vi "_ASIC_TEST_enlace.vi"(8 "error in":errorcluster, 11 "ftHandle_in":u32) -> (0 "error out":errorcluster, 3 "ftHandle_out":u32)   [LabVIEW 2009]
panel:
  out "Scaler 3 (20,21)":u16 format="%04x"
  out "Scaler 2 (18,19)":u16 format="%04x"
  out "Scaler 1 (16,17)":u16 format="%04x"
  out "Lectura asic (14,15)":u16 format="%04x"
  out "Vent. Sacaler (11,12,13)":u32 format="%06x"
  out "Periodo VGa (9,10)":u16 format="%04x"
  out "Pulse VGa (7,8)":u16 format="%04x"
  out "Ganacia VGA (6)":u8 format="%02x"
  out "adc (4,5)":u16 format="%04x"
  out "Asic (1,2,3)":u32 format="%06x"
  out "DIR 0 (CONFIG)":bool[](array[boolean])
  out "ERROR":bool
  out "DAC_IB":bool[](array[boolean])
  out "BUFF_ENA":bool
  out "LVDS_ENA1":bool
  out "LVDS_ENA0":bool
  out "MUX_ENA":string
  out "MUX_ENA#":i32
  out "IN 0":bool[](array[boolean])
  out "IN 6":bool[](array[boolean])
  out "IN 5":bool[](array[boolean])
  out "IN 4":bool[](array[boolean])
  out "IN 3":bool[](array[boolean])
  out "IN 2":bool[](array[boolean])
  out "IN 1":bool[](array[boolean])
  out "DAC_MUX#":i32
  out "DAC_MUX":string
  out "TH5":u16 format="%010b"
  out "TH4":u16 format="%010b"
  out "TH3":u16 format="%010b"
  out "TH2":u16 format="%010b"
  out "TH1":u16 format="%010b"
  out "TH0":u16 format="%010b"
  # "start vent. sca\nescribir ganancia\nactualizar pulso\nenable pulso\nstart tx asic\nreset asic\nescribir adc"
  # "Control_byte\nNum bit        Función\n0            \"Escribir\" ADC\n1                      \"INIT_R\" ASIC (reset)\n2                      \"start_tx\" ASIC para configuración ASIC\n3                      \"enable\" para el pulso\n4                      \"actualizar\" para el pulso\n5                      \"Escribir_ganancia\" para configuración ganancia\n6                      \"start\" para apertura ventana temportal scalers"
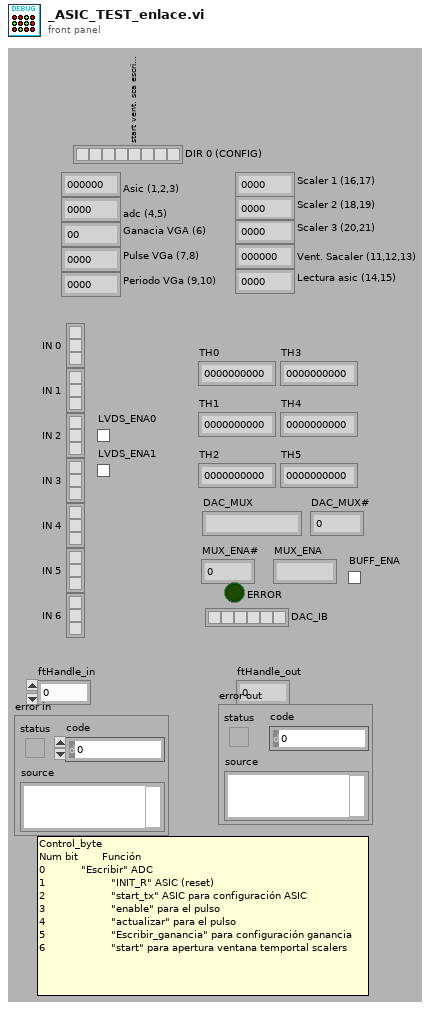
[diagram p1: front panel]
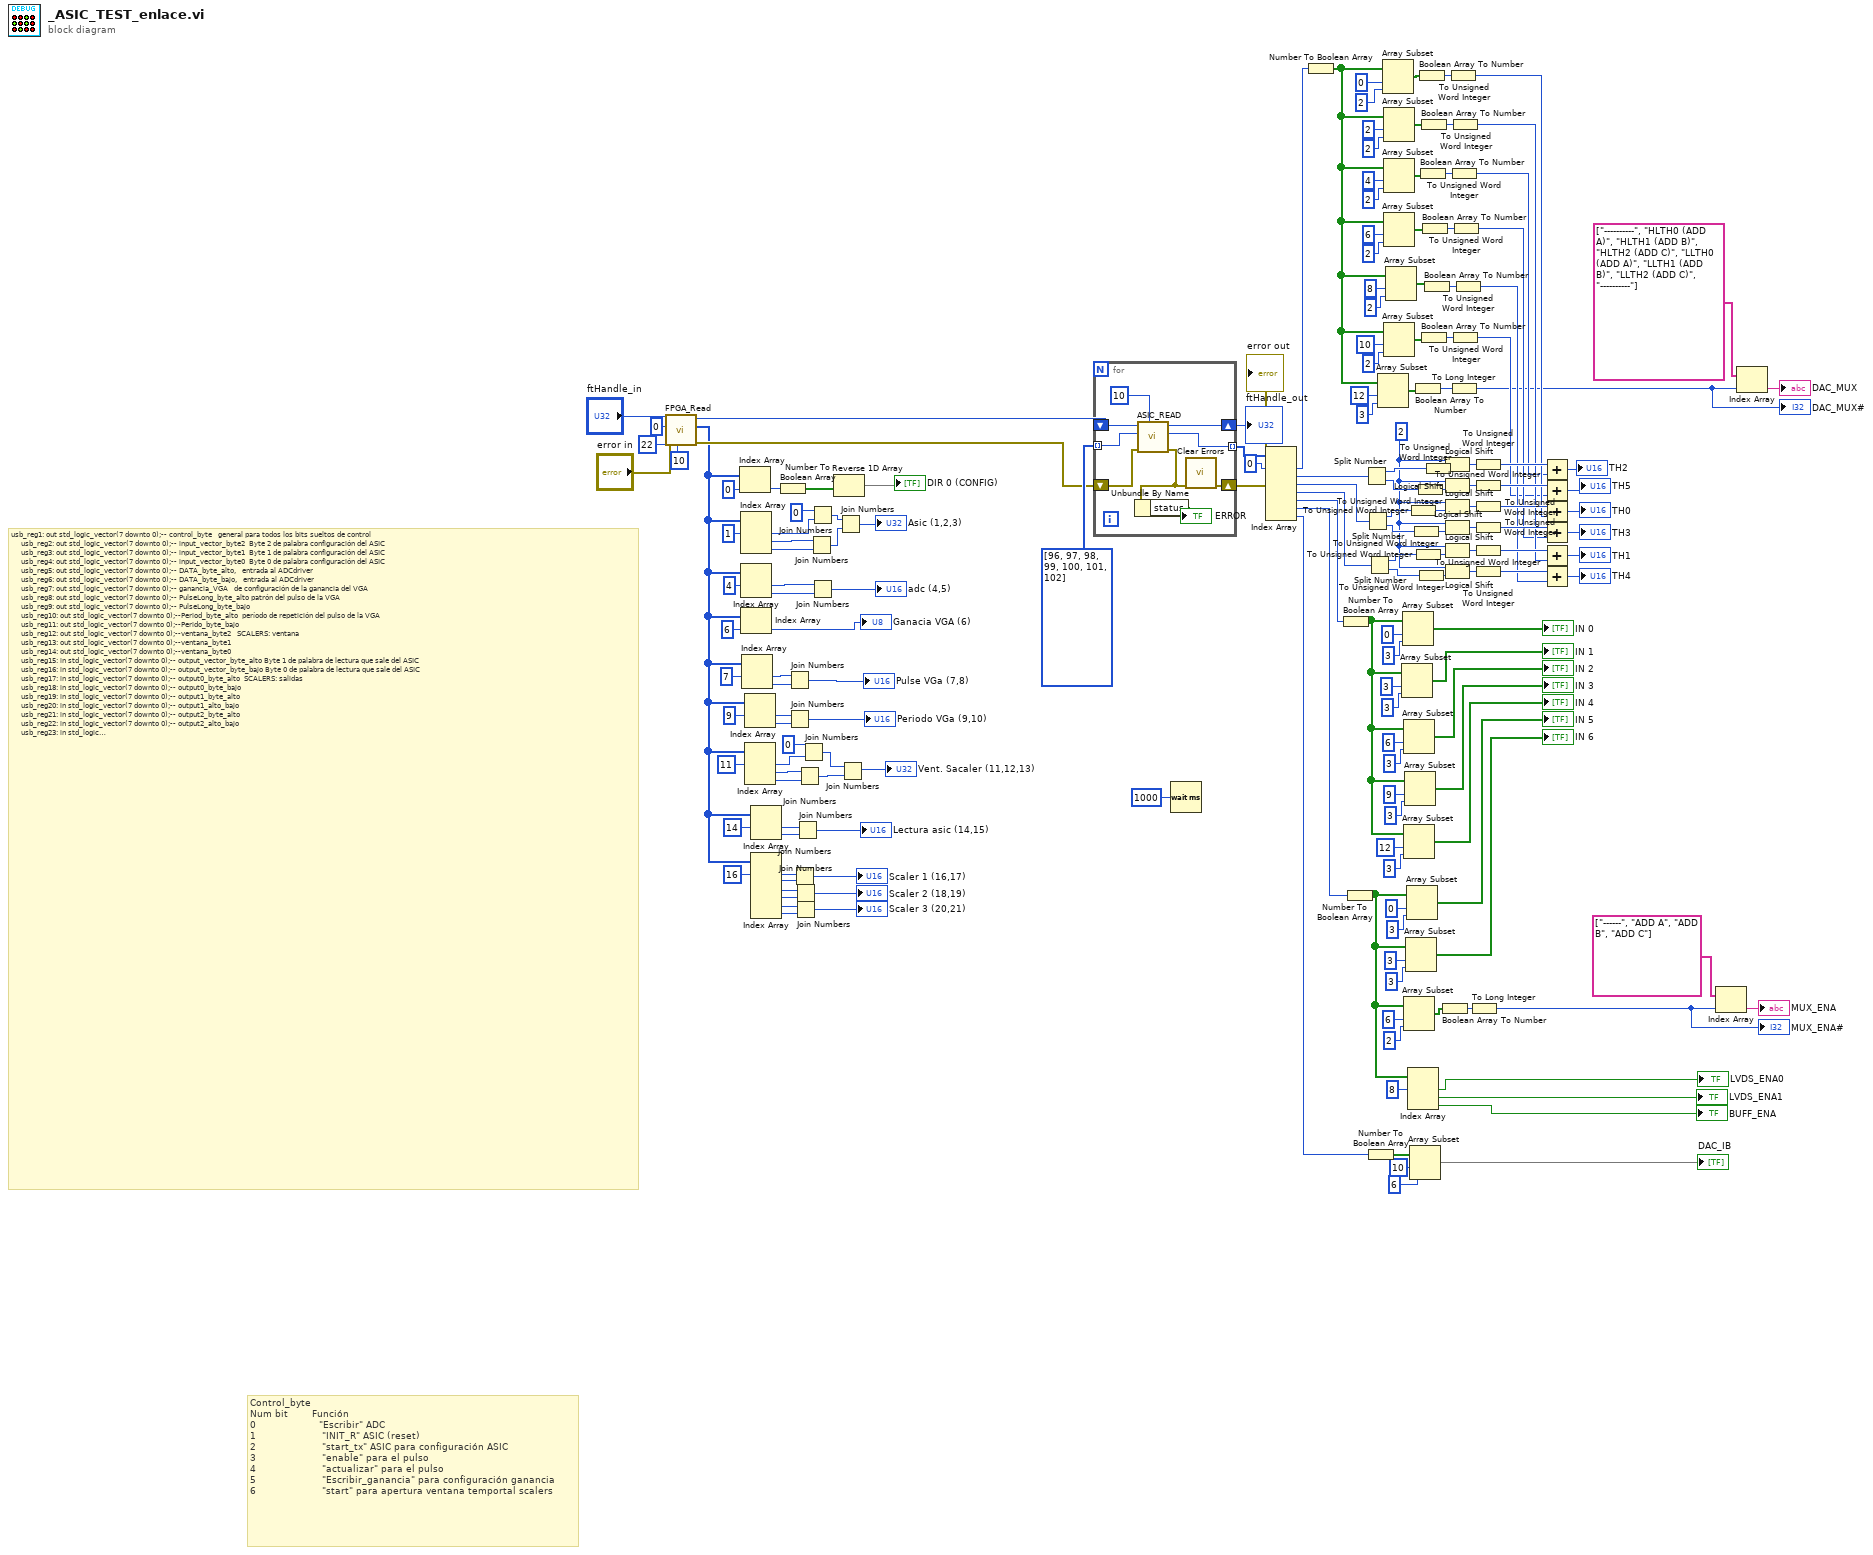
[diagram p0: block diagram]
diagram:
  w165 = i8 2 ("y")
  # "Control_byte\nNum bit        Función\n0                     \"Escribir\" ADC\n1                      \"INIT_R\" ASIC (reset)\n2                      \"start_tx\" ASIC para configuración ASIC\n3                      \"enable\" para el pulso\n4                      \"actualizar\" para el pulso\n5                      \"Escribir_ganancia\" para configuración ganancia\n6                      \"start\" para apertura ventana temportal scalers"
  # "usb_reg1: out std_logic_vector(7 downto 0);-- control_byte\t\t\tgeneral para todos los bits sueltos de control\n\t\t\t  usb_reg2: out std_logic_vector(7 downto 0);-- input_vector_byte2 \tByte 2 de palabra configuración del ASIC\n\t\t\t  usb_reg3: out std_logic_vector(7 downto 0);-- input_vector_byte1 \tByte 1 de palabra configuración del ASIC\n\t\t\t  usb_reg4: out std_logic_vector(7 downto 0);-- input_vector_byte0 \tByte 0 de palabra configuración del ASIC\n\t\t\t  usb_reg5: out std_logic_vector(7 downto 0);-- DATA_byte_alto, \t\tentrada al ADCdriver\n\t\t\t  usb_reg6: out std_logic_vector(7 downto 0);-- DATA_byte_bajo, \t\tentrada al ADCdriver\n\t\t\t  usb_reg7: out std_logic_vector(7 downto 0);-- ganancia_VGA\t\t\tde configuración de la ganancia del VGA\n\t\t\t  usb_reg8: out std_logic_vector(7 downto 0);-- PulseLong_byte_alto\tpatrón del pulso de la VGA\n\t\t\t  usb_reg9: out std_logic_vector(7 downto 0);-- PulseLong_byte_bajo\n\t\t\t  usb_reg10: out std_logic_vector(7 downto 0);--Period_byte_alto\t\tperíodo de repetición del pulso de la VGA\n\t\t\t  usb_reg11: out std_logic_vector(7 downto 0);--Perido_byte_bajo\n\t\t\t  usb_reg12: out std_logic_vector(7 downto 0);--ventana_byte2\t\t\tSCALERS: ventana\n\t\t\t  usb_reg13: out std_logic_vector(7 downto 0);--ventana_byte1\t\n\t\t\t  usb_reg14: out std_logic_vector(7 downto 0);--ventana_byte0\n\t\t\t  usb_reg15: in std_logic_vector(7 downto 0);-- output_vector_byte_alto\tByte 1 de palabra de lectura que sale del ASIC\n\t\t\t  usb_reg16: in std_logic_vector(7 downto 0);-- output_vector_byte_bajo\tByte 0 de palabra de lectura que sale del ASIC\n\t\t\t  usb_reg17: in std_logic_vector(7 downto 0);-- output0_byte_alto\t\tSCALERS: salidas\n\t\t\t  usb_reg18: in std_logic_vector(7 downto 0);-- output0_byte_bajo\n\t\t\t  usb_reg19: in std_logic_vector(7 downto 0);-- output1_byte_alto\n\t\t\t  usb_reg20: in std_logic_vector(7 downto 0);-- output1_alto_bajo \n\t\t\t  usb_reg21: in std_logic_vector(7 downto 0);-- output2_byte_alto \n\t\t\t  usb_reg22: in std_logic_vector(7 downto 0);-- output2_alto_bajo \n\t\t\t  usb_reg23: in std_logic_vector(7 downto 0);-- para el canal_0 del ADCdriver\n\t\t\t  usb_reg24: in std_logic_vector(7 downto 0);\n\t\t\t  usb_reg25: in std_logic_vector(7 downto 0);-- para el canal_1 del ADCdriver\n\t\t\t  usb_reg26: in std_logic_vector(7 downto 0);\n\t\t\t  usb_reg27: in std_logic_vector(7 downto 0);-- para el canal_2 del ADCdriver\n\t\t\t  usb_reg28: in std_logic_vector(7 downto 0);\n\t\t\t  usb_reg29: in std_logic_vector(7 downto 0);-- para el canal_3 del ADCdriver\n\t\t\t  usb_reg30: in std_logic_vector(7 downto 0);\n\t\t\t  usb_reg31: in std_logic_vector(7 downto 0);-- para el canal_4 del ADCdriver\n\t\t\t  usb_reg32: in std_logic_vector(7 downto 0);\n\t\t\t  usb_reg33: in std_logic_vector(7 downto 0);-- para el canal_5 del ADCdriver\n\t\t\t  usb_reg34: in std_logic_vector(7 downto 0);\n\t\t\t  usb_reg35: in std_logic_vector(7 downto 0);-- para el canal_6 del ADCdriver\n\t\t\t  usb_reg36: in std_logic_vector(7 downto 0);\n\t\t\t  usb_reg37: in std_logic_vector(7 downto 0);-- para el canal_7 del ADCdriver\n\t\t\t  usb_reg38: in std_logic_vector(7 downto 0);\n\t\t\t  usb_reg39: in std_logic_vector(7 downto 0);-- para el canal_8 del ADCdriver\n\t\t\t  usb_reg40: in std_logic_vector(7 downto 0);\n\t\t\t  usb_reg41: in std_logic_vector(7 downto 0);-- para el canal_9 del ADCdriver\n\t\t\t  usb_reg42: in std_logic_vector(7 downto 0);\n\t\t\t  usb_reg43: in std_logic_vector(7 downto 0);-- para el canal_10 del ADCdriver\n\t\t\t  usb_reg44: in std_logic_vector(7 downto 0)--;"
  n1 = call "FPGA_Read.vi"("Espera acceso USB"=u32 10, "error in"="error in", "Numero Bytes"=u8 22, "Dirección base"=u8 0, "ftHandle_in"="ftHandle_in") -> ("error out"=w56:errorcluster, "lpBuffer_out"=w15:u8[], "ftHandle_out"=w58:u32)  [unwired: 2 in, 2 out]
  n2 = Index Array(array=w15, index=0) -> (element=w37:u8)
  n3 = Index Array(array=w15, index #1=1 ("index")) -> (element #1=w32:u8, element #2=w33:u8, element #3=w34:u8)  [unwired: 2 in]
  n4 = Index Array(array=w15, index #1=4 ("index")) -> (element #1=w31:u8, element #2=w30:u8)  [unwired: 1 in]
  n5 = Index Array(array=w15, index=6) -> (element=→"Ganacia VGA (6)":u8)
  n6 = Index Array(array=w15, index #1=7 ("index")) -> (element #1=w24:u8, element #2=w25:u8)  [unwired: 1 in]
  n7 = Index Array(array=w15, index #1=9 ("index")) -> (element #1=w22:u8, element #2=w23:u8)  [unwired: 1 in]
  n8 = Index Array(array=w15, index #1=11 ("index")) -> (element #1=w18:u8, element #2=w16:u8, element #3=w17:u8)  [unwired: 2 in]
  n9 = Index Array(array=w15, index #1=14 ("index")) -> (element #1=w14:u8, element #2=w13:u8)  [unwired: 1 in]
  n10 = Index Array(array=w15, index #1=16 ("index")) -> (element #1=w11:u8, element #2=w10:u8, element #3=w8:u8, element #4=w7:u8, element #5=w6:u8, element #6=w5:u8)  [unwired: 5 in]
  n11 = Number To Boolean Array(number=w37) -> (Boolean array=w39:bool[])
  n12 = Join Numbers(hi=w24, lo=w25) -> ((hi.lo)=→"Pulse VGa (7,8)":u16)
  n13 = Join Numbers(hi=w22, lo=w23) -> ((hi.lo)=→"Periodo VGa (9,10)":u16)
  n14 = Join Numbers(hi=w11, lo=w10) -> ((hi.lo)=→"Scaler 1 (16,17)":u16)
  n15 = Join Numbers(hi=w8, lo=w7) -> ((hi.lo)=→"Scaler 2 (18,19)":u16)
  n16 = Join Numbers(hi=w6, lo=w5) -> ((hi.lo)=→"Scaler 3 (20,21)":u16)
  n17 = Join Numbers(hi=w14, lo=w13) -> ((hi.lo)=→"Lectura asic (14,15)":u16)
  n18 = Join Numbers(hi=w16, lo=w17) -> ((hi.lo)=w48:u16)
  n19 = Join Numbers(hi=u8 0, lo=w18) -> ((hi.lo)=w42:u16)
  n20 = Join Numbers(hi=w33, lo=w34) -> ((hi.lo)=w53:u16)
  n21 = Join Numbers(hi=u8 0, lo=w32) -> ((hi.lo)=w52:u16)
  n22 = Join Numbers(hi=w31, lo=w30) -> ((hi.lo)=→"adc (4,5)":u16)
  n23 = Reverse 1D Array(array=w39) -> (reversed array=→"DIR 0 (CONFIG)":bool[])
  n24 = Join Numbers(hi=w52, lo=w53) -> ((hi.lo)=→"Asic (1,2,3)":u32)
  n25 = Join Numbers(hi=w42, lo=w48) -> ((hi.lo)=→"Vent. Sacaler (11,12,13)":u32)
  n26 = for {
    tunnel: u8[] [96, 97, 98, 99, 100, 101, 102] -> [w183] mode=indexing
    tunnel: [w181] -> w175 mode=indexing
    shift-right: [w182] -> w2
    shift-left: w58 -> [w185]
    shift-right: [w180] -> w1
    shift-left: w56 -> [w179]
    n27 = call "ASIC_READ.vi"("Espera acceso USB"=u32 10, "error in"=w179, "Direccion Registro Asic"=w183, "ftHandle_in"=w185) -> ("error out"=w178:errorcluster, "Valor Asic"=w181:u16, "ftHandle_out"=w182:u32)  [unwired: 5 in]
    n28 = Unbundle By Name(w178) -> ("status"=→"ERROR":bool)
    n29 = call <vilib>:"Clear Errors.vi"("error in (no error)"=w178) -> ("error out"=w180:errorcluster)  [unwired: 6 in]
  }
  "ftHandle_out" <- w2
  "error out" <- w1
  n30 = Wait (ms)(milliseconds to wait=u32 1000) -> ()  [unwired: 1 out]
  n31 = Index Array(array=w175, index #1=0 ("index")) -> (element #1=w107:u16, element #2=w116:u16, element #3=w173:u16, element #4=w172:u16, element #5=w106:u16, element #6=w85:u16, element #7=w69:u16)  [unwired: 6 in]
  n32 = Number To Boolean Array(number=w107) -> (Boolean array=w111:bool[])
  n33 = Number To Boolean Array(number=w106) -> (Boolean array=w94:bool[])
  n34 = Number To Boolean Array(number=w85) -> (Boolean array=w75:bool[])
  n35 = Split Number(x=w116) -> (hi(x)=w171:u8, lo(x)=w170:u8)
  n36 = Split Number(x=w173) -> (hi(x)=w169:u8, lo(x)=w168:u8)
  n37 = Split Number(x=w172) -> (hi(x)=w167:u8, lo(x)=w166:u8)
  n38 = Number To Boolean Array(number=w69) -> (Boolean array=w70:bool[])
  n39 = Array Subset(array=w111, index=12, length=3) -> (w115:bool[])
  n40 = Array Subset(array=w111, index=0, length=2) -> (w162:bool[])
  n41 = Array Subset(array=w111, index=2, length=2) -> (w143:bool[])
  n42 = Array Subset(array=w111, index=4, length=2) -> (w141:bool[])
  n43 = Array Subset(array=w111, index=6, length=2) -> (w139:bool[])
  n44 = Array Subset(array=w111, index=10, length=2) -> (w135:bool[])
  n45 = Array Subset(array=w111, index=8, length=2) -> (w137:bool[])
  n46 = Array Subset(array=w94, index=3, length=3) -> (→"IN 1":bool[])
  n47 = Array Subset(array=w94, index=0, length=3) -> (→"IN 0":bool[])
  n48 = Array Subset(array=w94, index=6, length=3) -> (→"IN 2":bool[])
  n49 = Array Subset(array=w94, index=12, length=3) -> (→"IN 4":bool[])
  n50 = Array Subset(array=w75, index=6, length=2) -> (w78:bool[])
  n51 = Array Subset(array=w94, index=9, length=3) -> (→"IN 3":bool[])
  n52 = Array Subset(array=w75, index=3, length=3) -> (→"IN 6":bool[])
  n53 = Array Subset(array=w75, index=0, length=3) -> (→"IN 5":bool[])
  n54 = To Unsigned Word Integer(number=w169) -> (unsigned 16bit integer=w61:u16)
  n55 = Index Array(array=w75, index #1=8 ("index")) -> (element #1=→"LVDS_ENA0":bool, element #2=→"LVDS_ENA1":bool, element #3=→"BUFF_ENA":bool)  [unwired: 2 in]
  n56 = Array Subset(array=w70, index=10, length=6) -> (→"DAC_IB":bool[])
  n57 = To Unsigned Word Integer(number=w168) -> (unsigned 16bit integer=w62:u16)
  n58 = Boolean Array To Number(Boolean array=w115) -> (number=w114:u32)
  n59 = To Unsigned Word Integer(number=w167) -> (unsigned 16bit integer=w63:u16)
  n60 = To Unsigned Word Integer(number=w170) -> (unsigned 16bit integer=w60:u16)
  n61 = To Unsigned Word Integer(number=w166) -> (unsigned 16bit integer=w64:u16)
  n62 = Boolean Array To Number(Boolean array=w162) -> (number=w160:u32)
  n63 = Boolean Array To Number(Boolean array=w141) -> (number=w142:u32)
  n64 = Boolean Array To Number(Boolean array=w143) -> (number=w144:u32)
  n65 = Boolean Array To Number(Boolean array=w135) -> (number=w136:u32)
  n66 = Boolean Array To Number(Boolean array=w139) -> (number=w140:u32)
  n67 = Boolean Array To Number(Boolean array=w137) -> (number=w138:u32)
  n68 = To Unsigned Word Integer(number=w171) -> (unsigned 16bit integer=w59:u16)
  n69 = Boolean Array To Number(Boolean array=w78) -> (number=w77:u32)
  n70 = Logical Shift(y=w165, x=w59) -> (x << y=w161:u16)
  n71 = Logical Shift(y=w165, x=w60) -> (x << y=w158:u16)
  n72 = Logical Shift(y=w165, x=w61) -> (x << y=w134:u16)
  n73 = Logical Shift(y=w165, x=w62) -> (x << y=w133:u16)
  n74 = Logical Shift(y=w165, x=w63) -> (x << y=w132:u16)
  n75 = Logical Shift(y=w165, x=w64) -> (x << y=w131:u16)
  n76 = To Unsigned Word Integer(number=w160) -> (unsigned 16bit integer=w122:u16)
  n77 = To Unsigned Word Integer(number=w142) -> (unsigned 16bit integer=w120:u16)
  n78 = To Long Integer(number=w114) -> (32bit integer=w109:i32)
  "DAC_MUX#" <- w109
  n79 = To Unsigned Word Integer(number=w144) -> (unsigned 16bit integer=w121:u16)
  n80 = To Unsigned Word Integer(number=w136) -> (unsigned 16bit integer=w117:u16)
  n81 = To Unsigned Word Integer(number=w140) -> (unsigned 16bit integer=w119:u16)
  n82 = To Unsigned Word Integer(number=w138) -> (unsigned 16bit integer=w118:u16)
  n83 = To Long Integer(number=w77) -> (32bit integer=w76:i32)
  "MUX_ENA#" <- w76
  n84 = To Unsigned Word Integer(number=w161) -> (unsigned 16bit integer=w159:u16)
  n85 = To Unsigned Word Integer(number=w158) -> (unsigned 16bit integer=w157:u16)
  n86 = To Unsigned Word Integer(number=w134) -> (unsigned 16bit integer=w130:u16)
  n87 = To Unsigned Word Integer(number=w133) -> (unsigned 16bit integer=w129:u16)
  n88 = To Unsigned Word Integer(number=w132) -> (unsigned 16bit integer=w128:u16)
  n89 = To Unsigned Word Integer(number=w131) -> (unsigned 16bit integer=w127:u16)
  n90 = Add(x=w159, y=w120) -> (x+y=→"TH2":u16)
  n91 = Add(x=w157, y=w117) -> (x+y=→"TH5":u16)
  n92 = Add(x=w130, y=w122) -> (x+y=→"TH0":u16)
  n93 = Add(x=w129, y=w119) -> (x+y=→"TH3":u16)
  n94 = Add(x=w128, y=w121) -> (x+y=→"TH1":u16)
  n95 = Add(x=w127, y=w118) -> (x+y=→"TH4":u16)
  n96 = Index Array(array=string[] ["------", "ADD A", "ADD B", "ADD C"], index=w76) -> (element=→"MUX_ENA":string)
  n97 = Index Array(array=string[] ["----------", "HLTH0 (ADD A)", "HLTH1 (ADD B)", "HLTH2 (ADD C)", "LLTH0 (ADD A)", "LLTH1 (ADD B)", "LLTH2 (ADD C)", "----------"], index=w109) -> (element=→"DAC_MUX":string)
